vi "Mean (DBL) with Error Clusters.vi"(0 "x":dbl[](array[numeric]), 11 "error in":errorcluster) -> (4 "mean":dbl, 15 "error out":errorcluster)   [LabVIEW 2020]
doc: "This VI returns the mean of the input array using the standard LabVIEW analysis library, but accepts and returns error clusters."
uses:
  <vilib>/Analysis/baseanly.llb/Mean (DBL).vi
  <vilib>/Analysis/NI_AALBase.lvlib
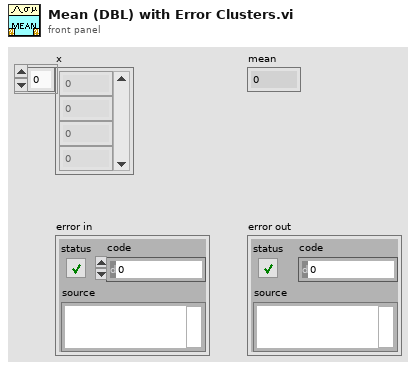
[diagram p1: front panel]
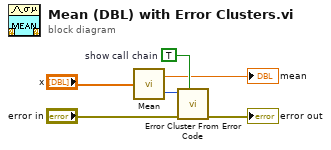
[diagram p0: block diagram]
diagram:
  w4 = TRUE  # show call chain
  n1 = call-poly <vilib>:"Mean.vi"("X"="x") -> ("mean"=→"mean":dbl, "error"=w3:i32)
  n2 = call <vilib>:"Error Cluster From Error Code.vi"("show call chain? (False)"=w4, "error in (no error)"="error in", "error code (0)"=w3) -> ("error out"=→"error out":errorcluster)  [unwired: 6 in]
